vi "CRYSet Main Generator Array.vi"(11 "Gen Idx":i32) -> (3 "Is Main?":bool)   [LabVIEW 2013]
uses:
  CRYMisc vis settings global.vi
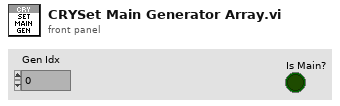
[diagram p1: front panel]
types:
  T1 = cluster{"Gen Idx":i32, "Chn Idx":i32, "Data":sgl[]}[]
  T2 = cluster{"Gen Idx":i32, "Chn Idx":i32, "Data":sgl[]}
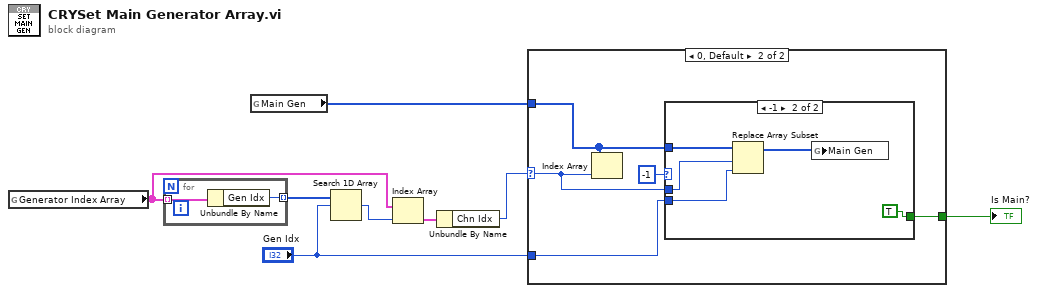
[diagram p0: block diagram]
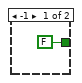
[diagram p2: hidden frame]
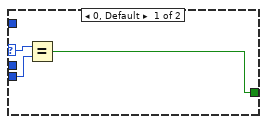
[diagram p3: hidden frame]
diagram:
  n1 = global read "CRYMisc vis settings global.vi" "Generator Index Array"() -> (w3:T1)
  n2 = for {
    tunnel: w3 -> [w10] mode=indexing
    tunnel: [w9] -> w6 mode=indexing
    n3 = Unbundle By Name(w10) -> ("Gen Idx"=w9:i32)
  }
  n4 = global read "CRYMisc vis settings global.vi" "Main Gen"() -> (w7:i32[])
  n5 = Search 1D Array(1D array=w6, element="Gen Idx") -> (index of element=w4:i32)  [unwired: 1 in]
  n6 = Index Array(array=w3, index=w4) -> (element=w2:T2)
  n7 = Unbundle By Name(w2) -> ("Chn Idx"=w1:i32)
  n8 = case shown="0, Default" w1 {
    selector: w1 -> [_ w13]
    tunnel: [FALSE w16] -> w8
    tunnel: w7 -> [_ w15]
    tunnel: "Gen Idx" -> [_ w14]
    frame -1 {
    }
    frame 0, Default {
      n9 = Index Array(array=w15, index=w13) -> ()  [unwired: 1 out]
      n10 = case shown="-1" -1 ("Numeric") {
        selector: -1 ("Numeric") -> [w19 _]
        tunnel: [w17 TRUE] -> w16
        tunnel: w15 -> [_ w23]
        tunnel: w14 -> [w18 w21]
        tunnel: w13 -> [_ w22]
        frame 0, Default {
          n11 = Equal?(x=w19, y=w18) -> (x = y?=w17:bool)
        }
        frame -1 {
          n12 = Replace Array Subset(array=w23, new element=w21, index=w22) -> (w20:i32[])
          n13 = global write "CRYMisc vis settings global.vi" "Main Gen"(w20) -> ()
        }
      }
    }
  }
  "Is Main?" <- w8
